vi "View.vi"(8 "error in (no error)":errorcluster, 11 "Customer In":refnum<class "Customer.lvclass">) -> (0 "error out":errorcluster, 3 "Customer Out":refnum<class "Customer.lvclass">)   [LabVIEW 2020, in "Customer.lvclass"]
doc: "This VI implements the main UI of the process. A reference to this VI should be set using the Set View VI Reference.vi method when the VI is started."
uses:
  Customer.lvclass
  C:/Program Files (x86)/National Instruments/LabVIEW 2020/vi.lib/Asteme/Triarc Framework/Process/Process.lvclass
  C:/Program Files (x86)/National Instruments/LabVIEW 2020/vi.lib/Asteme/Triarc Framework/View/View.lvclass
  Support/Beverages/TypeDefs/Drink Type.ctl
  Support/Beverages/TypeDefs/Options.ctl
  <vilib>/Asteme/Triarc Framework/View/View.lvclass/View.ctl
  Public/Order State.ctl
  <vilib>/Asteme/Triarc Framework/View/View.lvclass
  <vilib>/Asteme/Triarc Framework/Process/Process.lvclass
  Support/Beverages/Beverage/Beverage.lvclass
panel:
  out "All Items Received":bool
  out "Order in progress":bool
  out "Items Ordered":u32
  out "Items Received":u32
  out "Items Picked Up":string
  out "Price":dbl
  out "Order Number":u32
  in  "Reset Order":bool
  in  "Make Order":bool
  in  "Order":cluster{"Drink type":T1, "Options":T2[]}[](array[cluster])
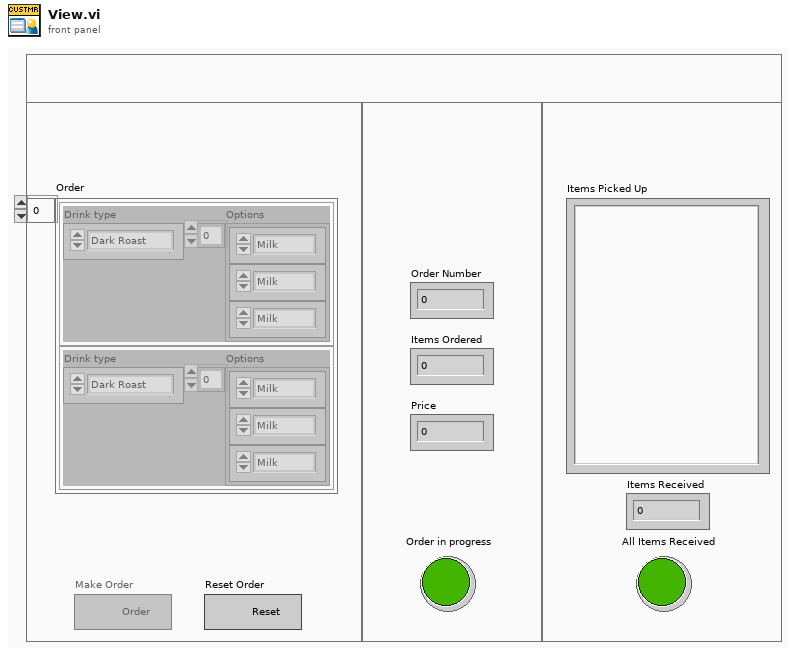
[diagram p1: front panel]
types:
  T1 = typedef "Beverage.lvclass/Drink Type.ctl" = enum16{"Dark Roast", "Decaf", "Espresso", "House Blend"}
  T2 = typedef "Beverage.lvclass/Options.ctl" = enum16{"<None>", "Milk", "Mocha", "Soy", "Whip"}
  T3 = enum8{"Enabled", "Disabled", "Disabled and Grayed Out"}
  T4 = typedef "Customer.lvclass/Order State.ctl" = cluster{"Order In Progress?":bool, "Order Number":u32, "Order Price":dbl, "Items Ordered":u32, "Items Received":u32, "Items Picked Up":string}
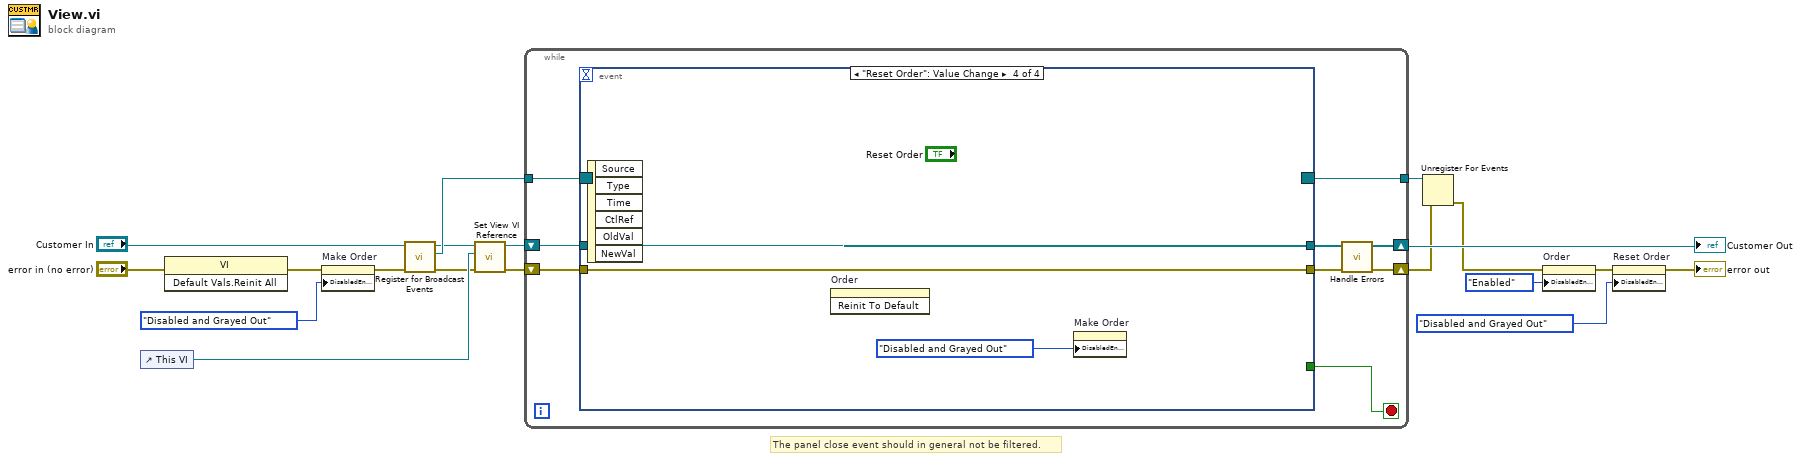
[diagram p0: block diagram]
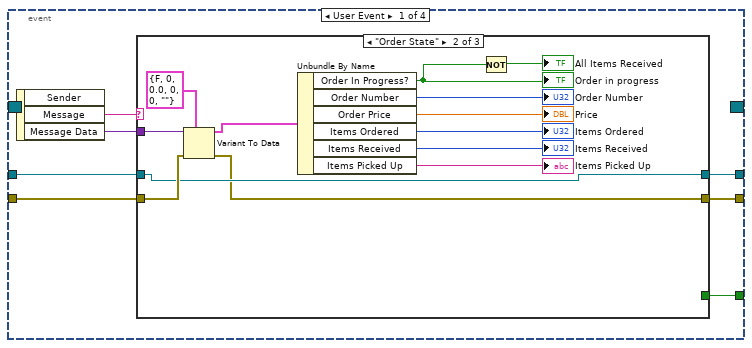
[diagram p2: hidden frame]
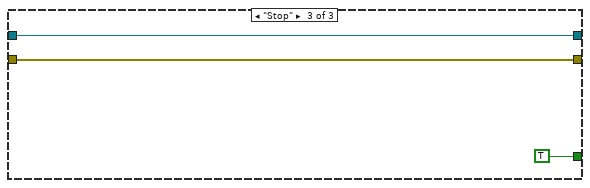
[diagram p4: hidden frame]
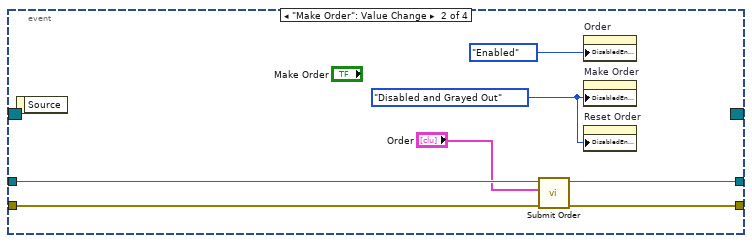
[diagram p5: hidden frame]
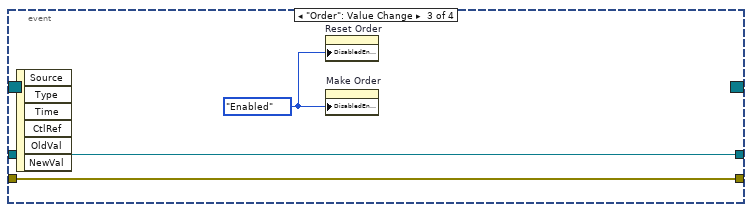
[diagram p6: hidden frame]
diagram:
  # "The panel close event should in general not be filtered."
  n1 = control-ref of="This VI"() -> (w17:refnum<vi>)
  n2 = invoke on="Invoke Node" class="VI" method="Default Vals.Reinit All"(error in="error in (no error)") -> (error out=w1:errorcluster)  [unwired: 2 in, 2 out]
  n3 = property on="Make Order" class="Bool"(error in=w1, "DisabledEnum"=T3."Disabled and Grayed Out" ("Disabled")) -> (error out=w8:errorcluster)  [unwired: 1 in, 1 out]
  n4 = call <vilib>:"Register for Broadcast Events.vi"("error in (no error)"=w8, "Process In"="Customer In") -> ("error out"=w15:errorcluster, "Event Registration Refnum Out"=w16:refnum<event-registration>, "Process Out"=w14:refnum<class "Customer.lvclass">)  [unwired: 7 in]
  n5 = call <vilib>:"Set View VI Reference.vi"("error in (no error)"=w15, "View VI Reference"=w17, "UI View in"=w14) -> ("error out"=w13:errorcluster, "UI View out"=w12:refnum<class "Customer.lvclass">)  [unwired: 7 in]
  n6 = while {
    shift-right: [w22] -> w19
    shift-left: w12 -> [w28]
    shift-right: [w20] -> w11
    shift-left: w13 -> [w26]
    tunnel: w16 -> [w25]
    tunnel: [w24] -> w10
    stop <- w23 stop-if-true
    n7 = event shown="[3] \"Reset Order\": Value Change" {
      selector: w25 -> [_ _ _ _]
      dyn-events: [_ _ _ _] -> w24
      timeout: _ -> [_ _ _ _]
      tunnel: w28 -> [w35 w57 w63 w66]
      tunnel: [w34 w58 w63 w66] -> w27
      tunnel: w26 -> [w32 w59 w62 w65]
      tunnel: [w33 w60 w62 w65] -> w21
      tunnel: [w30 _ _ _] -> w23
      event User Event {
        n8 = event-data() -> ("Message"=w31:string, "Message Data"=w29:variant)  [unwired: 1 in, 1 out]
        n9 = case shown="\"Order State\"" w31 {
          tunnel: w35 -> [w37 w40 w53]
          tunnel: [w37 w40 w53] -> w34
          tunnel: [w36 w39 w52] -> w33
          tunnel: w32 -> [w36 w49 w52]
          tunnel: [_ _ TRUE] -> w30
          tunnel: w29 -> [_ w50 _]
          frame Default {
          }
          frame "Order State" {
            n10 = Variant To Data(error in=w49, type=T4 {"Order In Progress?"=FALSE, "Order Number"=0, "Order Price"=0.0, "Items Ordered"=0, "Items Received"=0, "Items Picked Up"=""} ("Order State"), Variant=w50) -> (data=w38:T4, error out=w39:errorcluster)
            n11 = Unbundle By Name(w38) -> ("Order In Progress?"=w45:bool, "Order Number"=→"Order Number":u32, "Order Price"=→"Price":dbl, "Items Ordered"=→"Items Ordered":u32, "Items Received"=→"Items Received":u32, "Items Picked Up"=→"Items Picked Up":string)
            "Order in progress" <- w45
            n12 = Not(x=w45) -> (.not. x?=→"All Items Received":bool)
          }
          frame "Stop" {
          }
        }
      }
      event "Make Order": Value Change {
        w55 = T3."Disabled and Grayed Out" ("Disabled")
        n13 = event-data() -> ()  [unwired: 1 in, 1 out]
        n14 = call "Submit Order.vi"("error in (no error)"=w59, "Order Content"="Order", "Customer In"=w57) -> ("error out"=w60:errorcluster, "Customer Out"=w58:refnum<class "Customer.lvclass">)  [unwired: 7 in]
        n15 = property on="Order" class="Arr (strict)"("DisabledEnum"=T3."Enabled" ("Disabled")) -> ()  [unwired: 2 in, 2 out]
        n16 = property on="Make Order" class="Bool"("DisabledEnum"=w55) -> ()  [unwired: 2 in, 2 out]
        n17 = property on="Reset Order" class="Bool"("DisabledEnum"=w55) -> ()  [unwired: 2 in, 2 out]
      }
      event "Order": Value Change {
        w61 = T3."Enabled" ("Disabled")
        n18 = event-data() -> ()  [unwired: 1 in, 6 out]
        n19 = property on="Reset Order" class="Bool"("DisabledEnum"=w61) -> ()  [unwired: 2 in, 2 out]
        n20 = property on="Make Order" class="Bool"("DisabledEnum"=w61) -> ()  [unwired: 2 in, 2 out]
      }
      event "Reset Order": Value Change {
        n21 = event-data() -> ()  [unwired: 1 in, 6 out]
        n22 = invoke on="Order" class="Arr (strict)" method="Reinit To Default"() -> ()  [unwired: 3 in, 3 out]
        n23 = property on="Make Order" class="Bool"("DisabledEnum"=T3."Disabled and Grayed Out" ("Disabled")) -> ()  [unwired: 2 in, 2 out]
      }
    }
    n24 = call-dynamic "Handle Errors.vi"("error in (no error)"=w21, "Process In"=w27) -> ("error out"=w20:errorcluster, "Process Out"=w22:refnum<class "Customer.lvclass">)  [unwired: 8 in]
  }
  "Customer Out" <- w19
  n25 = Unregister For Events(event registration refnum=w10, error in=w11) -> (error out=w4:errorcluster)
  n26 = property on="Order" class="Arr (strict)"(error in=w4, "DisabledEnum"=T3."Enabled" ("Disabled")) -> (error out=w5:errorcluster)  [unwired: 1 in, 1 out]
  n27 = property on="Reset Order" class="Bool"(error in=w5, "DisabledEnum"=T3."Disabled and Grayed Out" ("Disabled")) -> (error out=→"error out":errorcluster)  [unwired: 1 in, 1 out]
